vi "IsDeviceValid.vi"(8 "error in (no error)":errorcluster caption="错误输入（无错误）", 10 "DeviceInd":u32, 11 "type":u16(ring)=2 items=["USB-CAN"=2, "USB-CAN2.0"=3]) -> (0 "error out":errorcluster caption="错误输出", 3 "Valid":bool)   [LabVIEW 2011]
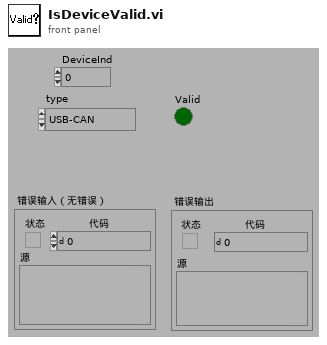
[diagram p1: front panel]
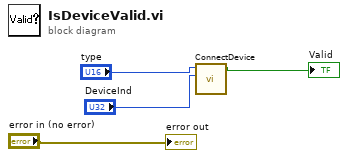
[diagram p0: block diagram]
diagram:
  n1 = call "ConnectDevice.vi"("DeviceInd"="DeviceInd", "type"="type") -> ("success"=→"Valid":bool)  [unwired: 8 in, 1 out]
  "error out" <- "error in (no error)"
